vi "Read Key (Boolean).vi"(7 "section":string, 8 "error in (no error)":errorcluster, 9 "default value":bool, 10 "key":string, 11 "refnum":T1) -> (0 "error out":errorcluster, 1 "value":bool, 2 "found?":bool, 3 "refnum out":T1)   [LabVIEW 2009]
doc: "Reads a value associated with a key in a specified section from the configuration data identified by <B>refnum</B>. If the key does not exist, the VI returns the default value. You can use this polymorphic VI to read the following types of values from a key: Boolean, double-precision numeric, signed integer, path, string, and unsigned integer. The data type you wire to the <B>default value</B> input determines the polymorphic instance to use."
uses:
  <vilib>/Utility/config.llb/Config Data RefNum.ctl
  <vilib>/Utility/config.llb/NI_LVConfig.lvlib
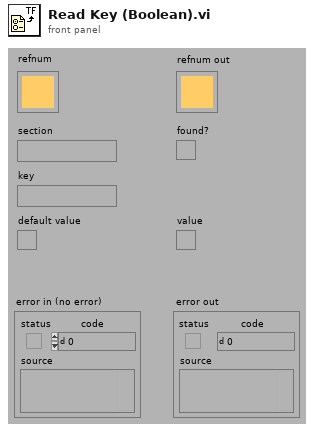
[diagram p1: front panel]
types:
  T1 = typedef "NI_LVConfig.lvlib/Config Data RefNum.ctl" = refnum<k1>
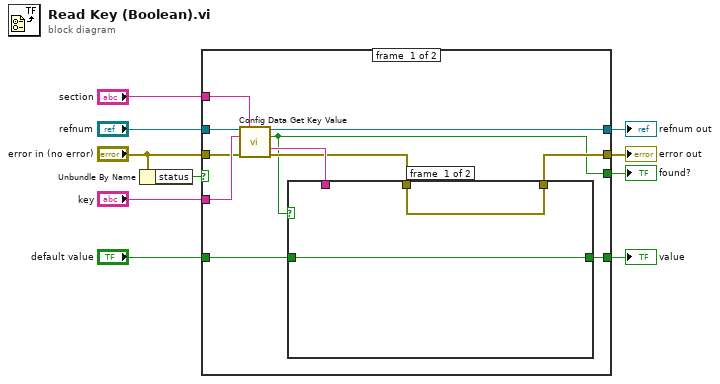
[diagram p0: block diagram]
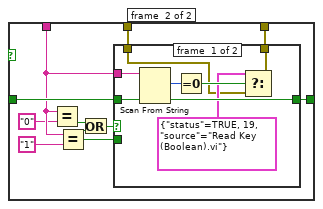
[diagram p2: hidden frame]
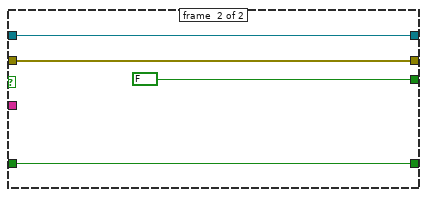
[diagram p4: hidden frame]
diagram:
  n1 = Unbundle By Name("error in (no error)") -> ("status"=w10:bool)
  n2 = case shown="False" w10 {
    tunnel: [w18 w46] -> w4
    tunnel: [w12 w47] -> w1
    tunnel: "refnum" -> [w16 w46]
    tunnel: "error in (no error)" -> [w17 w47]
    tunnel: "section" -> [w21 _]
    tunnel: "key" -> [w20 _]
    tunnel: [w11 FALSE ("section exists?")] -> w3
    tunnel: [w19 w45] -> w2
    tunnel: "default value" -> [w15 w45]
    frame #0 {
      n3 = call "Config Data Get Key Value.vi"("config data"=w16, "section"=w21, "key"=w20, "error in (no error)"=w17) -> ("config data out"=w18:T1, "key exists?"=w11:bool, "key value"=w14:string, "error out"=w13:errorcluster)  [unwired: 6 in, 2 out]
      n4 = case shown="True" w11 {
        tunnel: [w23 w33] -> w19
        tunnel: w15 -> [w23 w32]
        tunnel: w14 -> [_ w31]
        tunnel: w13 -> [w22 w25]
        tunnel: [w22 w24] -> w12
        frame #0 {
        }
        frame #1 {
          n5 = Equal?(x=w31, y="0") -> (x = y?=w27:bool)
          n6 = Equal?(x=w31, y="1") -> (x = y?=w28:bool)
          n7 = Or(x=w27, y=w28) -> (x .or. y?=w26:bool)
          n8 = case shown="False" w26 {
            tunnel: [w41 w43] -> w33
            tunnel: w31 -> [w40 _]
            tunnel: w32 -> [w39 _]
            tunnel: w28 -> [_ w43]
            tunnel: w25 -> [w34 w42]
            tunnel: [w36 w42] -> w24
            frame #0 {
              n9 = Scan From String(input string=w40, default 1=w39) -> (offset past scan=w38:u32, output 1=w41:bool)  [unwired: 3 in, 2 out]
              n10 = Equal To 0?(x=w38) -> (x = 0?=w37:bool)
              n11 = Select(t=cluster{"status":bool, u16, "source":string} {"status"=TRUE, 19, "source"="Read Key (Boolean).vi"} ("f"), s=w37, f=w34) -> (s? t:f=w36:errorcluster)
            }
            frame #1 {
            }
          }
        }
      }
    }
    frame #1 {
    }
  }
  "error out" <- w1
  "refnum out" <- w4
  "value" <- w2
  "found?" <- w3
